vi "test_Setup_Device_Connection.vi"(8 "error in (no error)":errorcluster, 10 "device selection":enum16{"monochromator", "CCD", "SCD"}(ring), 11 "set-up a connection":bool) -> (0 "error out":errorcluster, 1 "Monochromator out":refnum<class "Monochromator.lvclass">, 2 "CCD out":refnum<class "CCD.lvclass">, 3 "SCD out":refnum<class "SCD.lvclass">)   [LabVIEW 2023]
uses:
  Classes/Mono/Monochromator.lvclass
  Classes/CCD/CCD.lvclass
  Classes/SCD/SCD.lvclass
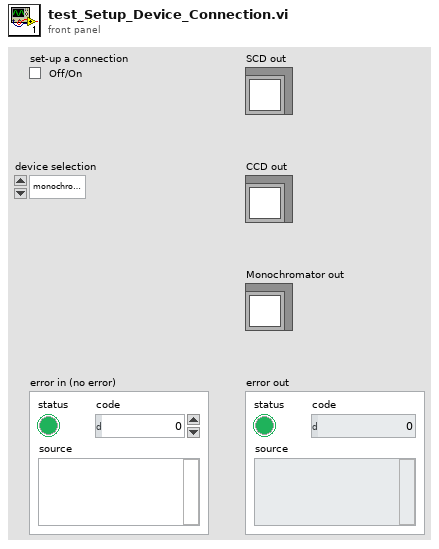
[diagram p1: front panel]
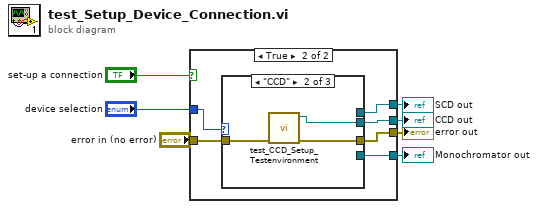
[diagram p0: block diagram]
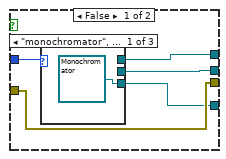
[diagram p2: hidden frame]
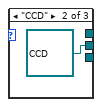
[diagram p3: hidden frame]
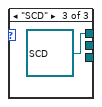
[diagram p4: hidden frame]
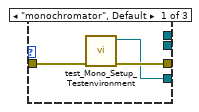
[diagram p5: hidden frame]
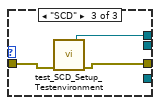
[diagram p6: hidden frame]
diagram:
  n1 = case shown="True" "set-up a connection" {
    tunnel: "error in (no error)" -> [w12 w21]
    tunnel: [w12 w20] -> w2
    tunnel: [w11 w16] -> w4
    tunnel: [w10 w19] -> w5
    tunnel: [w9 w17] -> w6
    tunnel: "device selection" -> [w8 w18]
    frame False {
      n2 = case shown="\"monochromator\", Default" w8 {
        tunnel: [refnum<class "Monochromator.lvclass"> refnum ("Monochromator.lvclass") _ _] -> w11
        tunnel: [_ refnum<class "CCD.lvclass"> refnum ("CCD in") _] -> w10
        tunnel: [_ _ refnum<class "SCD.lvclass"> refnum ("SCD.lvclass")] -> w9
        frame "monochromator", Default {
        }
        frame "CCD" {
        }
        frame "SCD" {
        }
      }
    }
    frame True {
      n3 = case shown="\"CCD\"" w18 {
        tunnel: w21 -> [w24 w27 w30]
        tunnel: [w23 w26 w29] -> w20
        tunnel: [_ w25 _] -> w19
        tunnel: [_ _ w28] -> w17
        tunnel: [w22 _ _] -> w16
        frame "monochromator", Default {
          n4 = call "test_Mono_Setup_Testenvironment.vi"("error in"=w24) -> ("error out"=w23:errorcluster, "Monochromator out"=w22:refnum<class "Monochromator.lvclass">)  [unwired: 8 in, 1 out]
        }
        frame "CCD" {
          n5 = call "test_CCD_Setup_Testenvironment.vi"("error in"=w27) -> ("error out"=w26:errorcluster, "CCD out"=w25:refnum<class "CCD.lvclass">)  [unwired: 8 in, 1 out]
        }
        frame "SCD" {
          n6 = call "test_SCD_Setup_Testenvironment.vi"("error in"=w30) -> ("error out"=w29:errorcluster, "SCD out"=w28:refnum<class "SCD.lvclass">)  [unwired: 8 in, 1 out]
        }
      }
    }
  }
  "SCD out" <- w6
  "CCD out" <- w5
  "Monochromator out" <- w4
  "error out" <- w2
